vi "Import Parameters Configuration to New AIM MIL-STD-1553 Custom Device.vi"() -> ()   [LabVIEW 2020]
uses:
  AIM MIL-STD-1553 Scripting Example Support.lvlib
  <vilib>/addons/VeriStand Custom Device Scripting APIs/AIM MIL-STD-1553/Shared/Initialization Method.ctl
  <vilib>/addons/VeriStand Custom Device Scripting APIs/AIM MIL-STD-1553/Shared/Device Parameters.ctl
  NationalInstruments.VeriStand.SystemDefinitionAPI
  <vilib>/addons/VeriStand Custom Device Scripting APIs/AIM MIL-STD-1553/Shared/Coupling Mode.ctl
  <vilib>/addons/VeriStand Custom Device Scripting APIs/AIM MIL-STD-1553/Shared/Bus Selection.ctl
panel:
  in  "Example Documentation":string="Overview: Demonstrates using the Ballard MIL-STD-1553 scripting API to configure the custom device by importing a parameters configuration file. \n\nInstructions:\n1. Specify the Custom Device Name and set the PXI Slot Number and Core Number for your Ballard hardware. \n2. Specify the Parameters Configuration File. This parameters configuration file must be consistent with the schema published on the GitHub repo: \nhttps://github.com/ni/niveristand-ballard-milStd1553-custom-device/blob/main/Docs/Parameters%20XML%20File/Parameters_XML_Schema.xsd\nFor successful deployment, the parameters configuration file must also be consistent with the hardware configuration file.\n3. Specify the Hardware Configuration File. The hardware configuration file must be consistent with the schema installed by the Ballard hardware driver at \nC:\\Program Files (x86)\\Astronics Ballard Technology LabVIEW Driver\\Help\\index.html.\n4. (VeriStand) Optionally, to perform avionics bus communications with Ballard MIL-STD-1553 hardware you may:\n   a. Open the Ballard MIL-STD-1553 System Definition in VeriStand.\n   b. Configure the PXI Linux RT Target.\n   c. Deploy the scripted system definition."
  in  "Core Number":i32
  in  "PXI Slot Number":i32=2
  in  "Custom Device Name":string="Ballard MIL-STD-1553"
  in  "Parameters Configuration File":path=path "Support/VeriStand MIL-STD-1553 Parameters.xml"
  in  "Hardware Configuration File":path=path "Support/Ballard MIL-STD-1553 Hardware.xml"
  in  "Base System Definition File":path=path "Support/Base.nivssdf"
  in  "Output System Definition File":path=path "Support/Imported Configuration Ballard MIL-STD-1553.nivssdf"
  out "Ballard MIL-STD-1553 System Definition":path
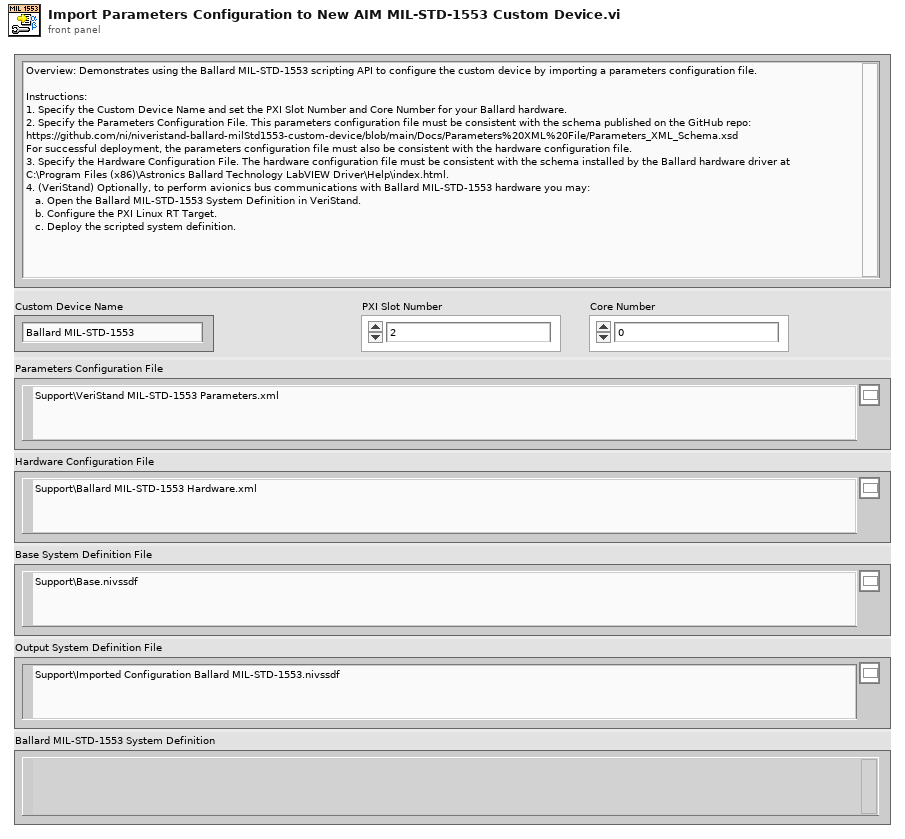
[diagram p1: front panel]
types:
  T1 = typedef "Device Parameters.ctl" = cluster{"initialization method":T2, "card number":i32, "pxi slot number":i32, "biu number":i32, "bus selection":T3, "coupling mode":T4}
  T2 = typedef "Initialization Method.ctl" = enum16{"PXI Slot Number", "Card Number"}
  T3 = typedef "Bus Selection.ctl" = enum16{"Both", "Primary", "Secondary"}
  T4 = typedef "Coupling Mode.ctl" = enum16{"Isolated Onboard Termination", "Transformer Coupled", "Direct Coupled", "External with Onboard Termination", "Onboard Digital Wrap-around"}
  T5 = typedef "Custom Device API.lvlib/Custom Device Item Ref.ctl" = u64
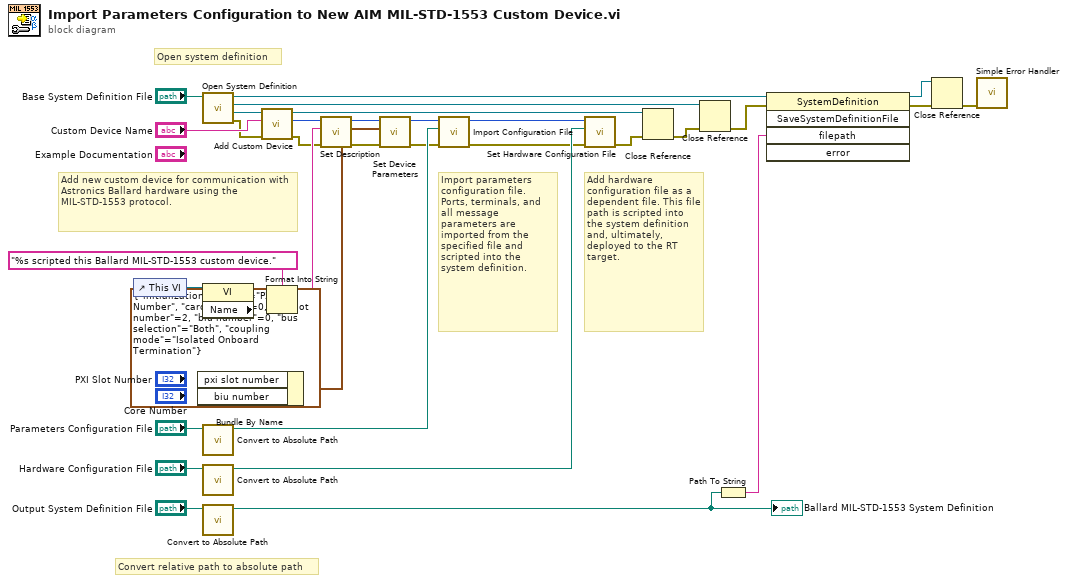
[diagram p0: block diagram]
diagram:
  # "Add hardware configuration file as a dependent file. This file path is scripted into the system definition and, ultimately, deployed to the RT target."
  # "Import parameters configuration file. Ports, terminals, and all message parameters are imported from the specified file and scripted into the system definition."
  # "Add new custom device for communication with Astronics Ballard hardware using the MIL-STD-1553 protocol."
  # "Convert relative path to absolute path"
  # "Open system definition"
  n1 = control-ref of="This VI"() -> (w14:refnum<vi>)
  n2 = Bundle By Name(cluster=T1 {"initialization method"=enum."PXI Slot Number", "card number"=0, "pxi slot number"=2, "biu number"=0, "bus selection"=enum."Both", "coupling mode"=enum."Isolated Onboard Termination"} ("device parameters"), "pxi slot number"="PXI Slot Number", "biu number"="Core Number") -> (w8:T1)
  n3 = call "Open System Definition.vi"("system definition file"="Base System Definition File") -> ("error out"=w16:errorcluster, "target"=w26:refnum<k24>, "root"=w18:refnum<k24>, "system definition"=w17:refnum<k24>)  [unwired: 7 in]
  n4 = property class="VI"(reference=w14) -> ("Name"=w13:string)  [unwired: 1 in, 2 out]
  n5 = call "Convert to Absolute Path.vi"("system definition file"="Parameters Configuration File") -> ("absolute path"=w24:path)  [unwired: 10 in]
  n6 = call "Convert to Absolute Path.vi"("system definition file"="Hardware Configuration File") -> ("absolute path"=w23:path)  [unwired: 10 in]
  n7 = call "Convert to Absolute Path.vi"("system definition file"="Output System Definition File") -> ("absolute path"=w22:path)  [unwired: 10 in]
  "Ballard MIL-STD-1553 System Definition" <- w22
  n8 = call <vilib>:"Add Custom Device.vi"("error in"=w16, "name"="Custom Device Name", "target in"=w26) -> ("error out"=w6:errorcluster, "Ballard MIL-STD 1553 custom device"=w5:T5, "target out"=w19:refnum<k24>)  [unwired: 6 in]
  n9 = Format Into String(format string="%s scripted this Ballard MIL-STD-1553 custom device." ("description"), w13) -> (resulting string=w12:string)  [unwired: 2 in, 1 out]
  n10 = call <vilib>:"Set Description.vi"("error in"=w6, "description"=w12, "Ballard MIL-STD 1553 custom device in"=w5) -> ("error out"=w3:errorcluster, "Ballard MIL-STD 1553 custom device out"=w4:T5)  [unwired: 7 in]
  n11 = call <vilib>:"Set Device Parameters.vi"("error in"=w3, "device parameters"=w8, "Ballard MIL-STD 1553 custom device in"=w4) -> ("error out"=w2:errorcluster, "Ballard MIL-STD 1553 custom device out"=w1:T5)  [unwired: 7 in]
  n12 = call <vilib>:"Import Configuration File.vi"("error in"=w2, "parameters configuration file path"=w24, "Ballard MIL-STD 1553 custom device in"=w1) -> ("error out"=w20:errorcluster, "Ballard MIL-STD 1553 custom device out"=w25:T5)  [unwired: 7 in]
  n13 = call <vilib>:"Set Hardware Configuration File.vi"("error in"=w20, "hardware configuration file path"=w23, "Ballard MIL-STD 1553 custom device in"=w25) -> ("error out"=w7:errorcluster)  [unwired: 7 in, 1 out]
  n14 = Close Reference(reference=w19, error in (no error)=w7) -> (error out=w29:errorcluster)
  n15 = Close Reference(reference=w18, error in (no error)=w29) -> (error out=w32:errorcluster)
  n16 = Path To String(path=w22) -> (string=w35:string)
  n17 = invoke class="SystemDefinition" method="SaveSystemDefinitionFile"(reference=w17, error in=w32, "filepath"=w35) -> (reference out=w33:refnum<k24>, error out=w34:errorcluster)  [unwired: 2 in, 3 out]
  n18 = Close Reference(reference=w33, error in (no error)=w34) -> (error out=w31:errorcluster)
  n19 = call <vilib>:"Simple Error Handler.vi"("error in (no error)"=w31) -> ()  [unwired: 1 in, 8 out]
